vi "Parse Refrigerant Mixture file_d.vi"(9 "Mixture File Path":path) -> (1 "Mixture Definition String":string, 2 "Mixture Name":string)   [LabVIEW 2017]
doc: "Reads the Refrigerant mixture file defined by the path and retruns the mixutre name as well as it's percent composition.\n\nDeveloped by:\nGreg Sussman\nProcess Automation Corp\nwww.processauto.com\n(267)685-1249"
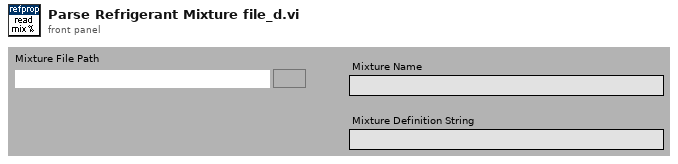
[diagram p1: front panel]
types:
  T1 = enum16{"open", "open or create", "create or replace", "create", "open (read only)"}
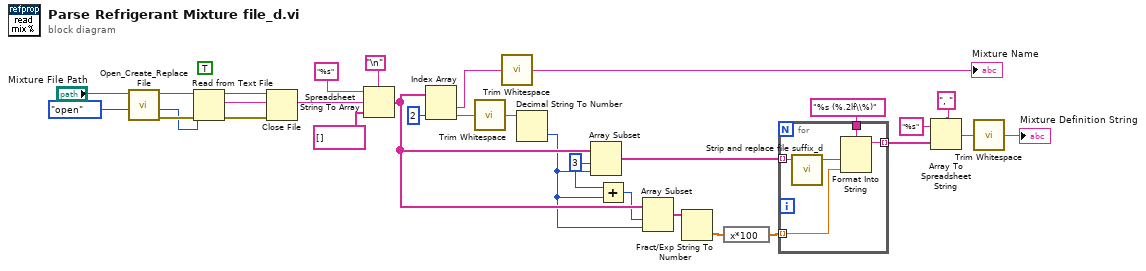
[diagram p0: block diagram]
diagram:
  (unwired) TRUE ("convert eol (F)")
  w23 = 3 ("index")
  n1 = call <vilib>:"Open_Create_Replace File.vi"("function (open:0)"=T1."open", "file path"="Mixture File Path") -> ("error out"=w5:errorcluster, "file size (bytes)"=w1:i32, "refnum"=w4:refnum<file>)  [unwired: 6 in, 1 out]
  n2 = Read from Text File(file (use dialog)=w4, count=w1, error in=w5) -> (refnum out=w2:refnum<file>, text=w12:string, error out=w3:errorcluster)  [unwired: 1 in, 1 out]
  n3 = Close File(refnum=w2, error in=w3) -> ()  [unwired: 2 out]
  n4 = Spreadsheet String To Array(delimiter (Tab)="\n", format string="%s", spreadsheet string=w12, array type (2D Dbl)=string[] []) -> (array=w24:string[])
  n5 = Index Array(array=w24, index #2=2 ("index")) -> (element #1=w10:string, element #2=w26:string)  [unwired: 1 in]
  n6 = call <vilib>:"Trim Whitespace.vi"("string"=w26) -> ("trimmed string"=w25:string)  [unwired: 1 in]
  n7 = call <vilib>:"Trim Whitespace.vi"("string"=w10) -> ("trimmed string"=→"Mixture Name":string)  [unwired: 1 in]
  n8 = Decimal String To Number(string=w25) -> (number=w21:i32)  [unwired: 2 in, 1 out]
  n9 = Array Subset(array=w24, index=w23, length=w21) -> (w20:string[])
  n10 = Add(x=w23, y=w21) -> (x+y=w22:i32)
  n11 = Array Subset(array=w24, index=w22, length=w21) -> (w19:string[])
  n12 = Fract/Exp String To Number(string=w19) -> (number=w13:dbl[])  [unwired: 3 in, 1 out]
  n13 = expression code="x*100"(w13) -> (w14:dbl[])
  n14 = for {
    tunnel: w20 -> [w35] mode=indexing
    tunnel: w14 -> [w33] mode=indexing
    tunnel: [w32] -> w18 mode=indexing
    tunnel: "%s (%.2lf\\%)" -> [w31]
    n15 = call "Strip and replace file suffix_d.vi"("File Name"=w35) -> ("File Name"=w34:string)  [unwired: 3 in, 1 out]
    n16 = Format Into String(format string=w31, w34, w33) -> (resulting string=w32:string)  [unwired: 2 in, 1 out]
  }
  n17 = Array To Spreadsheet String(delimiter (Tab)=", ", array=w18, 3:"%s" ("format string")) -> (spreadsheet string=w8:string)
  n18 = call <vilib>:"Trim Whitespace.vi"("string"=w8) -> ("trimmed string"=→"Mixture Definition String":string)  [unwired: 1 in]
